vi "Valve Type.vi"(11 "SequencedValves in":refnum<class "SequencedValves.lvclass">) -> (2 "Valve Type":string)   [LabVIEW 2020, in "VolatusControl.lvlib" / "SequencedValves.lvclass"]
uses:
  SequencedValves.lvclass
  SequencedValves.lvclass/SequencedValves.ctl
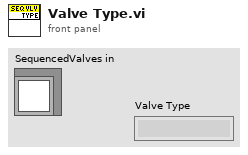
[diagram p1: front panel]
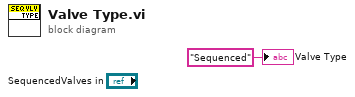
[diagram p0: block diagram]
diagram:
  "Valve Type" <- "Sequenced" ("Valve Type")
